vi "From JSON Text (Variant).vi"(7 "Data Type and Default Value":variant, 9 "error in (no error)":errorcluster, 10 "Offset":i32, 11 "JSON":string) -> (1 "error out":errorcluster, 3 "Variant out":variant)   [LabVIEW 2019, in "JSONtext.lvlib"]
doc: "Convert JSON to the Data Type entered, which may be a cluster or array."
uses:
  JSONtext.lvlib
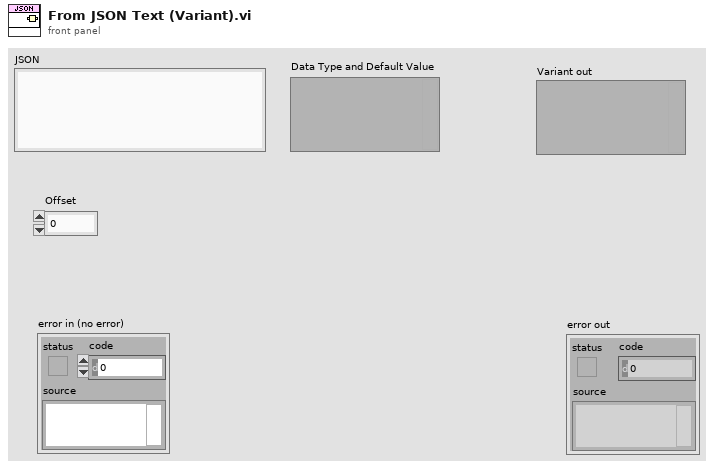
[diagram p1: front panel]
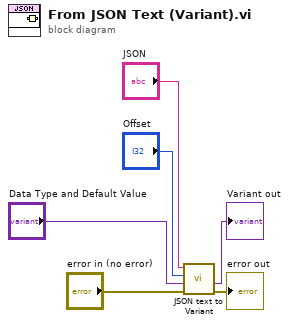
[diagram p0: block diagram]
diagram:
  n1 = call "JSON text to Variant.vi"("error in (no error)"="error in (no error)", "Data Type"="Data Type and Default Value", "Offset"="Offset", "JSON"="JSON") -> ("error out"=→"error out":errorcluster, "Variant out"=→"Variant out":variant)  [unwired: 6 in]
